vi "TestPointer.Clear Error.Null.vi"(8 "error in (no error)":errorcluster) -> (0 "error out":errorcluster, 3 "error cleared?":bool)   [LabVIEW 2016, in "TestPointer.lvclass"]
uses:
  TestPointer.lvclass
  Source/Classes/Pointer/Memory.Pointer.Errors.ctl
  Source/Classes/Pointer/Memory.Pointer.lvclass
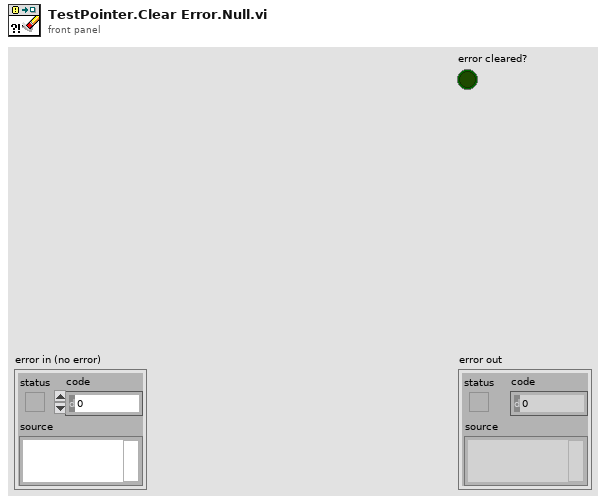
[diagram p1: front panel]
types:
  T1 = typedef "Memory Manager.lvlib/Memory.Pointer.lvclass/Memory.Pointer.Errors.ctl" = enum16{"No Error", "Null Pointer", "Out of Bounds", "Buffer Underflow", "Size Mismatch", "Zone"}
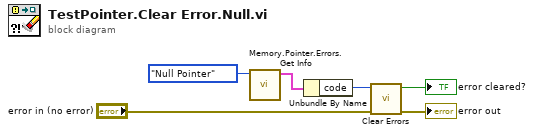
[diagram p0: block diagram]
diagram:
  n1 = call "Memory.Pointer.Errors.Get Info.vi"("error"=Memory.Pointer.Errors."Null Pointer") -> ("error info"=w3:cluster{"code":i32, "description":string})  [unwired: 10 in]
  n2 = Unbundle By Name(w3) -> ("code"=w6:i32)
  n3 = call <vilib>:"Clear Errors.vi"("error in (no error)"="error in (no error)", "specific error code to clear (0: all)"=w6) -> ("error out"=→"error out":errorcluster, "specific error cleared?"=→"error cleared?":bool)  [unwired: 4 in]
